vi "from_td_array.vi"(5 "type":refnum<class "TypeDescriptor.lvclass">, 8 "error in":errorcluster, 11 "type descriptor array":i16[](array[numeric])) -> (0 "error out":errorcluster, 3 "TypeDescriptor out":refnum<class "TypeDescriptor.lvclass">)   [LabVIEW 2020, in "lvdata.lvlib" / "type_descriptor.lvlib" / "TypeDescriptor.lvclass"]
uses:
  TypeDescriptor.lvclass
  C:/projects/OpenG-Variant-Data-Library/source/library/Bytes/Bytes.lvclass
  Type Descriptor Enumeration.ctl
  ArrayTD/Array.lvclass
  C:/projects/OpenG-Variant-Data-Library/source/library/LVData/Type Descriptor/TypeDescriptor.lvclass
  TypeDescriptor.lvclass/TypeDescriptor.ctl
  Bytes/Bytes.lvclass/Bytes.ctl
  Bytes/Bytes.lvclass
  openg_variant.lvlib
  C:/projects/OpenG-Variant-Data-Library/source/library/LVData/Type Descriptor/ArrayTD/Array.lvclass
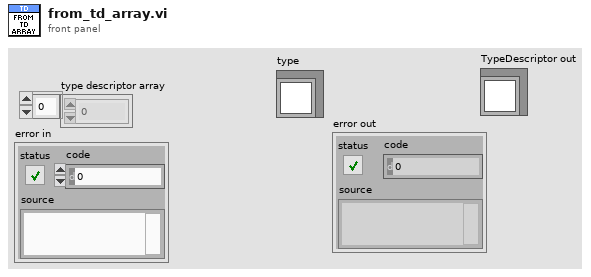
[diagram p1: front panel]
types:
  T1 = typedef "openg_variant.lvlib/Type Descriptor Enumeration.ctl" = enum8{"<Null>", "I8", "I16", "I32", "I64", "U8", "U16", "U32", "U64", "SGL", "DBL", "EXT", "CSG", "CDB", "CXT", "0x0F", "0x10", "0x11", "0x12", "0x13", "0x14", "Enum U8", "Enum U16", "Enum U32", "Enum U64", "SGL PQ", "DBL PQ", "EXT PQ", "CSG PQ", "CDB PQ", "CXT PQ", "0x1F", "0x20", "Boolean", "0x22", "0x23", "0x24", "0x25", "0x26", "0x27", "0x28", "0x29", "0x2A", "0x2B", "0x2C", "0x2D", "0x2E", "0x2F", "String", "0x31", "Path", "Pict", "0x34", "0x35", "0x36", "DAQ", "0x38", "0x39", "0x3A", "0x3B", "0x3C", "0x3D", "0x3E", "0x3F", "Array", "0x41", "0x42", "0x43", "0x44", "0x45", "0x46", "0x47", "0x48", "0x49", "0x4A", "0x4B", "0x4C", "0x4D", "0x4E", "0x4F", "Cluster", "0x51", "0x52", "Variant", "Waveform", "0x55", "0x56", "0x57", "0x58", "0x59", "0x5A", "0x5B", "0x5C", "0x5D", "0x5E", "Fixed Point", "0x60", "0x61", "0x62", "0x63", "0x64", "0x65", "0x66", "0x67", "0x68", "0x69", "0x6A", "0x6B", "0x6C", "0x6D", "0x6E", "0x6F", "Refnum", "0x71", "0x72", "Set Collection", "Map Collection"}
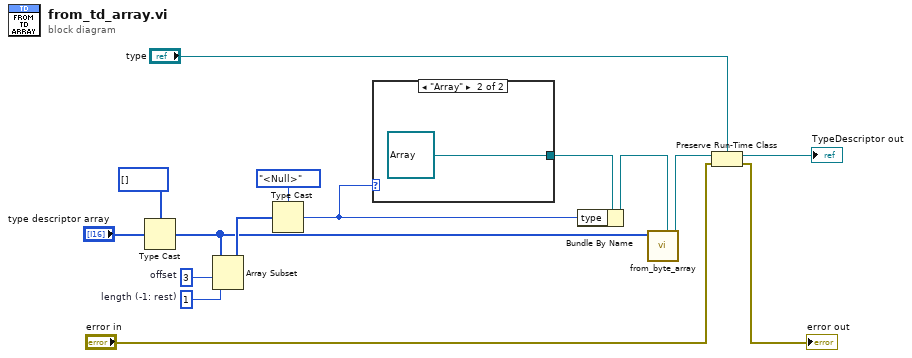
[diagram p0: block diagram]
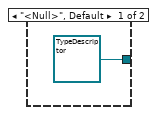
[diagram p2: hidden frame]
diagram:
  w10 = 1  # length (-1: rest)
  w11 = 3  # offset
  n1 = Type Cast(type=u8[] [] ("unsigned byte array"), x="type descriptor array") -> (*(type *) &x=w6:u8[])
  n2 = Array Subset(array=w6, index=w11, length=w10) -> (w7:u8[])
  n3 = Type Cast(type=Type_Descriptor_Enumeration."<Null>", x=w7) -> (*(type *) &x=w8:T1)
  n4 = case shown="\"Array\"" w8 {
    tunnel: [refnum<class "TypeDescriptor.lvclass"> refnum ("lvdata.lvlib:TypeDescriptor.lvclass") refnum<class "Array.lvclass"> refnum ("lvdata.lvlib:ArrayTD.lvclass")] -> w5
    frame "<Null>", Default {
    }
    frame "Array" {
    }
  }
  n5 = Bundle By Name(cluster=w5, "type"=w8) -> (w9:refnum<class "TypeDescriptor.lvclass">)
  n6 = call "from_byte_array.vi"("type"=w9, "unsigned byte array"=w6) -> ("Bytes out"=w15:refnum<class "TypeDescriptor.lvclass">)  [unwired: 9 in]
  n7 = Preserve Run-Time Class(object in=w15, error in="error in", 2:"type") -> (object out=→"TypeDescriptor out":refnum<class "TypeDescriptor.lvclass">, error out=→"error out":errorcluster)
